vi "read_subpanel_notifier.vi"(8 "error in (no error)":errorcluster, 11 "panel in":refnum<class "panel.lvclass">) -> (0 "error out":errorcluster, 2 "subpanel_notifier":refnum<notifier>, 3 "panel out":refnum<class "panel.lvclass">)   [LabVIEW 2015, in "panel.lvclass"]
uses:
  panel.lvclass
  panel.lvclass/panel.ctl
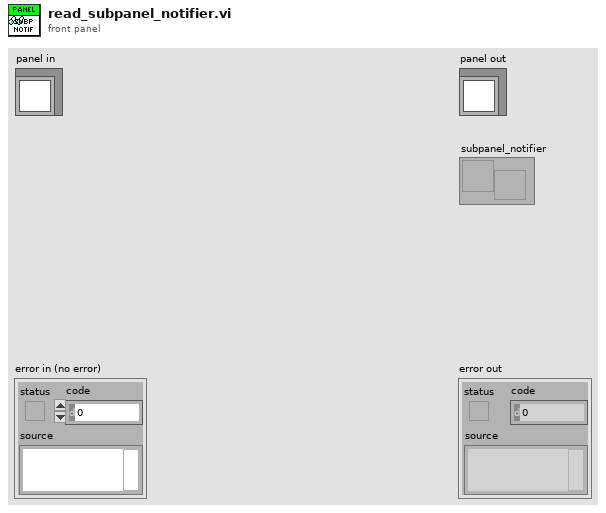
[diagram p1: front panel]
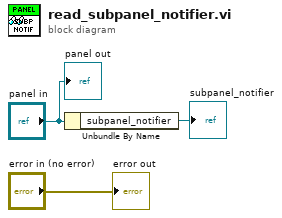
[diagram p0: block diagram]
diagram:
  n1 = Unbundle By Name("panel in") -> ("subpanel_notifier"=→"subpanel_notifier":refnum<notifier>)
  "error out" <- "error in (no error)"
  "panel out" <- "panel in"
